vi "Moving Average Half Center.vi"(10 "MA half size":i32=180, 11 "Data Array":dbl[](array[numeric])) -> (3 "Moving Average":dbl[](array[numeric]))   [LabVIEW 2016]
uses:
  <vilib>/Analysis/baseanly.llb/Mean (DBL).vi
  <vilib>/Analysis/NI_AALBase.lvlib
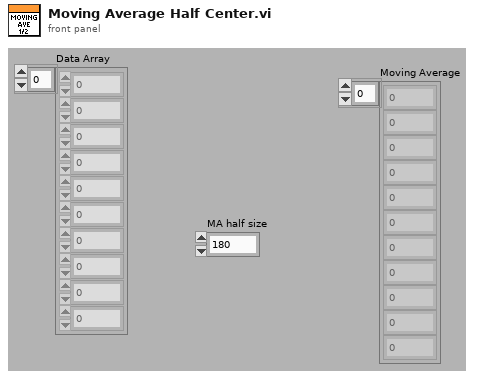
[diagram p1: front panel]
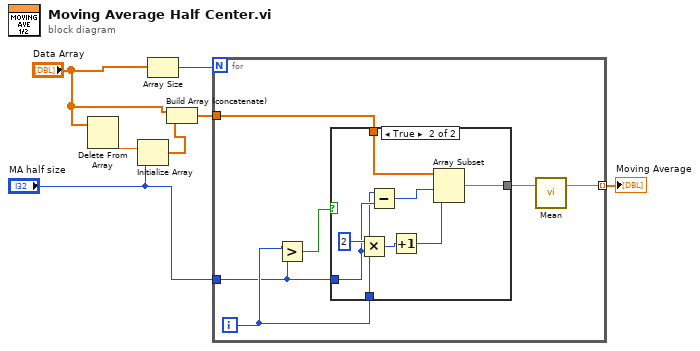
[diagram p0: block diagram]
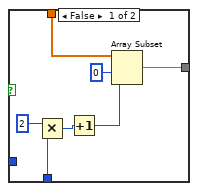
[diagram p2: hidden frame]
diagram:
  n1 = Delete From Array(array="Data Array") -> (deleted portion=w6:dbl)  [unwired: 2 in, 1 out]
  n2 = Initialize Array(w6, "MA half size") -> (w4:dbl[])
  n3 = Array Size(array="Data Array") -> (size(s)=w7:i32)
  n4 = Build Array (concatenate)("Data Array", w4) -> (w2:dbl[])
  n5 = for {
    N: w7 -> [_]
    tunnel: "MA half size" -> [w8]
    tunnel: w2 -> [w11]
    tunnel: [w9] -> w1 mode=indexing
    i -> [w12]
    n6 = Greater?(x=w12, y=w8) -> (0:w13:bool)
    n7 = case shown="True" w13 {
      tunnel: w12 -> [w20 w22]
      tunnel: w11 -> [w15 w25]
      tunnel: [w14 w24] -> w10
      tunnel: w8 -> [_ w23]
      frame False {
        n8 = Multiply(x=2, y=w20) -> (x*y=w18:i32)
        n9 = Increment(x=w18) -> (x+1=w17:i32)
        n10 = Array Subset(array=w15, index=0, length=w17) -> (w14:dbl[])
      }
      frame True {
        n11 = Multiply(x=2, y=w23) -> (x*y=w27:i32)
        n12 = Subtract(x=w22, y=w23) -> (x-y=w21:i32)
        n13 = Increment(x=w27) -> (x+1=w26:i32)
        n14 = Array Subset(array=w25, index=w21, length=w26) -> (w24:dbl[])
      }
    }
    n15 = call-poly <vilib>:"Mean.vi"("X"=w10) -> ("mean"=w9:dbl)  [unwired: 1 out]
  }
  "Moving Average" <- w1
